vi "tio32_TestBoardAvail.vi"(0 "VISA resource name":refnum<visa-resource-name>, 5 "device addess to check":i32=4660 format="%x", 11 "error in (no error)":errorcluster) -> (4 "VISA resource name out":refnum<visa-resource-name>, 6 "return":i32=666, 8 "device number result":i32=-1, 15 "error out":errorcluster)   [LabVIEW 2011]
uses:
  l_pse_dll/Tio32.dll
panel:
  # "tio32_TestBoardAvail"
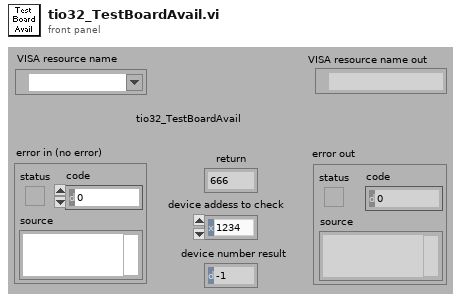
[diagram p1: front panel]
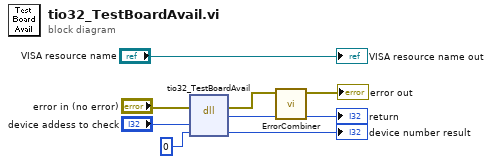
[diagram p0: block diagram]
diagram:
  n1 = dll-call lib="C:/Users/Ikaika's/Documents/DCC/Apps/INA231/INA231-SFT-rev1/INA231-Sourcecode-rev1/INA231/Shell Resources/l_pse_dll/Tio32.dll" fn="tio32_TestBoardAvail"(error in="error in (no error)", "adr"="device addess to check", "pAdr"=i16 0 ("pdevNo")) -> (error out=w2:errorcluster, "Rückgabetyp"=w3:i32, "pAdr"=→"device number result":i32)  [unwired: 3 in, 1 out]
  n2 = call "ErrorCombiner.vi"("Return In"=w3, "error in (no error)"=w2) -> ("Return Out"=→"return":i32, "error out"=→"error out":errorcluster)  [unwired: 8 in]
  "VISA resource name out" <- "VISA resource name"
